vi "log_event_queue.vi"(8 "error in":errorcluster) -> (0 "error out":errorcluster, 2 "Log event queue":refnum<queue>)   [LabVIEW 2013]
uses:
  log_event.ctl
panel:
  # "Get log_event queue for sending log events to logger.  Internal.  To receive events for logging or display, use log_event_notifier.vi"
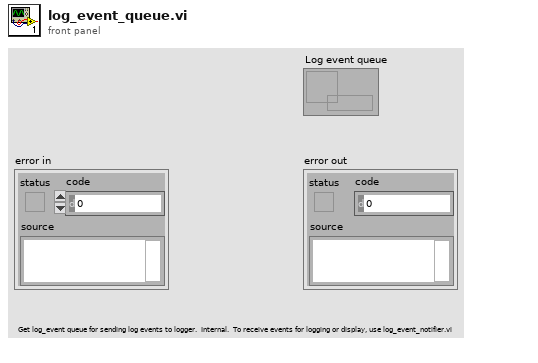
[diagram p1: front panel]
types:
  T1 = typedef "log_event.ctl" = cluster{"Facility ID":i32, "Severity":enum16{"OK", "Debug", "Warn", "Error"}, "Timestamp":timestamp, "Facility":string, "State":string, "Message":string}
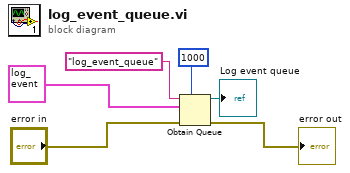
[diagram p0: block diagram]
diagram:
  n1 = Obtain Queue(max queue size (-1, unlimited)=1000, name (unnamed)="log_event_queue", element data type=T1 {"Facility ID"=0, "Severity"=enum."Debug", "Timestamp"=timestamp(0 s since 1904-01-01), "Facility"="", "State"="", "Message"=""} ("Log event"), error in (no error)="error in") -> (queue out=→"Log event queue":refnum<queue>, error out=→"error out":errorcluster)  [unwired: 1 in, 1 out]
